vi "Resize DI Command Array.vi"(1 "Command in":T1={"Mode"=enum."Off", "Digital Input"=enum."Unused", "Default Profile Index"=0, "Cal Freq [Hz]"=0.0, "Cal Duration [s]"=0.0, "Cal Increment [s]"=0.0, "Cal Pulses"=0, "TMP Command Sequence"=[{"Duration [s]"=0.0, "Level"=FALSE, "Run/Stop"=FALSE, "Profile Index"=0}, {"Duration [s]"=0.0, "Level"=FALSE, "Run/Stop"=FALSE, "Profile Index"=0}, {"Duration [s]"=0.0, "Level"=FALSE, "Run/Stop"=FALSE, "Profile Index"=0}, {"Duration [s]"=0.0, "Level"=FALSE, "Run/Stop"=FALSE, "Profile Index"=0}, {"Duration [s]"=0.0, "Level"=FALSE, "Run/Stop"=FALSE, "Profile Index"=0}, {"Duration [s]"=0.0, "Level"=FALSE, "Run/Stop"=FALSE, "Profile Index"=0}, {"Duration [s]"=0.0, "Level"=FALSE, "Run/Stop"=FALSE, "Profile Index"=0}, {"Duration [s]"=0.0, "Level"=FALSE, "Run/Stop"=FALSE, "Profile Index"=0}], "EPT TDC Offset [CAD]"=0.0, "EPT Window Start [DBTDC]"=0.0, "EPT Window End [DBTDC]"=0.0, "EPT Angles"=[{"Enable"=FALSE, "Timing [DBTDC]"=0.0, "Duration [s]"=0.0, "Profile Index"=0}, {"Enable"=FALSE, "Timing [DBTDC]"=0.0, "Duration [s]"=0.0, "Profile Index"=0}, {"Enable"=FALSE, "Timing [DBTDC]"=0.0, "Duration [s]"=0.0, "Profile Index"=0}, {"Enable"=FALSE, "Timing [DBTDC]"=0.0, "Duration [s]"=0.0, "Profile Index"=0}], "EPT Skip Fire"=FALSE, "EPT Skip Index"=0, "EPT Precharge Duration [s]"=0.0, "EPT Precharge Profile Index"=0} {"EPT Precharge Profile Index" max=15; "EPT Precharge Duration [s]" min=0 format="%#_4p"; "Default Profile Index" max=15; "Cal Increment [s]" format="%#_3p"; "TMP Command Sequence"."Profile Index" max=7; "TMP Command Sequence"."Duration [s]" min=0 max=100 format="%#_3p"; "Cal Pulses" max=511; "EPT Skip Index" max=7; "EPT Angles"."Profile Index" max=7; "EPT Angles"."Duration [s]" min=0 max=100 format="%#_3p"; "Cal Duration [s]" format="%#_3p"; "Cal Freq [Hz]" format="%#_3p"}) -> (0 "Command out":T1={"Mode"=enum."Off", "Digital Input"=enum."Unused", "Default Profile Index"=0, "Cal Freq [Hz]"=0.0, "Cal Duration [s]"=0.0, "Cal Increment [s]"=0.0, "Cal Pulses"=0, "TMP Command Sequence"=[{"Duration [s]"=0.0, "Level"=FALSE, "Run/Stop"=FALSE, "Profile Index"=0}, {"Duration [s]"=0.0, "Level"=FALSE, "Run/Stop"=FALSE, "Profile Index"=0}, {"Duration [s]"=0.0, "Level"=FALSE, "Run/Stop"=FALSE, "Profile Index"=0}, {"Duration [s]"=0.0, "Level"=FALSE, "Run/Stop"=FALSE, "Profile Index"=0}, {"Duration [s]"=0.0, "Level"=FALSE, "Run/Stop"=FALSE, "Profile Index"=0}, {"Duration [s]"=0.0, "Level"=FALSE, "Run/Stop"=FALSE, "Profile Index"=0}, {"Duration [s]"=0.0, "Level"=FALSE, "Run/Stop"=FALSE, "Profile Index"=0}, {"Duration [s]"=0.0, "Level"=FALSE, "Run/Stop"=FALSE, "Profile Index"=0}], "EPT TDC Offset [CAD]"=0.0, "EPT Window Start [DBTDC]"=0.0, "EPT Window End [DBTDC]"=0.0, "EPT Angles"=[{"Enable"=FALSE, "Timing [DBTDC]"=0.0, "Duration [s]"=0.0, "Profile Index"=0}, {"Enable"=FALSE, "Timing [DBTDC]"=0.0, "Duration [s]"=0.0, "Profile Index"=0}, {"Enable"=FALSE, "Timing [DBTDC]"=0.0, "Duration [s]"=0.0, "Profile Index"=0}, {"Enable"=FALSE, "Timing [DBTDC]"=0.0, "Duration [s]"=0.0, "Profile Index"=0}], "EPT Skip Fire"=FALSE, "EPT Skip Index"=0, "EPT Precharge Duration [s]"=0.0, "EPT Precharge Profile Index"=0} {"EPT Precharge Profile Index" max=15; "EPT Precharge Duration [s]" min=0 format="%#_4p"; "Default Profile Index" max=15; "Cal Increment [s]" format="%#_3p"; "TMP Command Sequence"."Profile Index" max=7; "TMP Command Sequence"."Duration [s]" min=0 max=100 format="%#_3p"; "Cal Pulses" max=511; "EPT Skip Index" max=7; "EPT Angles"."Profile Index" max=7; "EPT Angles"."Duration [s]" min=0 max=100 format="%#_3p"; "Cal Duration [s]" format="%#_3p"; "Cal Freq [Hz]" format="%#_3p"})   [LabVIEW 2016]
uses:
  <vilib>/Powertrain Controls/Device Drivers/DCM/DI/RT/Command.ctl
  <vilib>/Powertrain Controls/Device Drivers/DCM/DI/FPGA/Mode.ctl
  <vilib>/Powertrain Controls/Device Drivers/DCM/Rev0/FPGA/Digital Channel.ctl
  <vilib>/Powertrain Controls/Device Drivers/DCM/DI/RT/Command Sequence.ctl
  <vilib>/Powertrain Controls/Device Drivers/DCM/DI/RT/Angle Control.ctl
  <vilib>/Powertrain Controls/Device Drivers/DCM/DI/RT/DCM - RT - DI.lvlib
  <vilib>/Powertrain Controls/Device Drivers/DCM/DI/FPGA/DCM - FPGA - DI.lvlib
  <vilib>/Powertrain Controls/Device Drivers/DCM/Rev0/FPGA/DCM - FPGA.lvlib
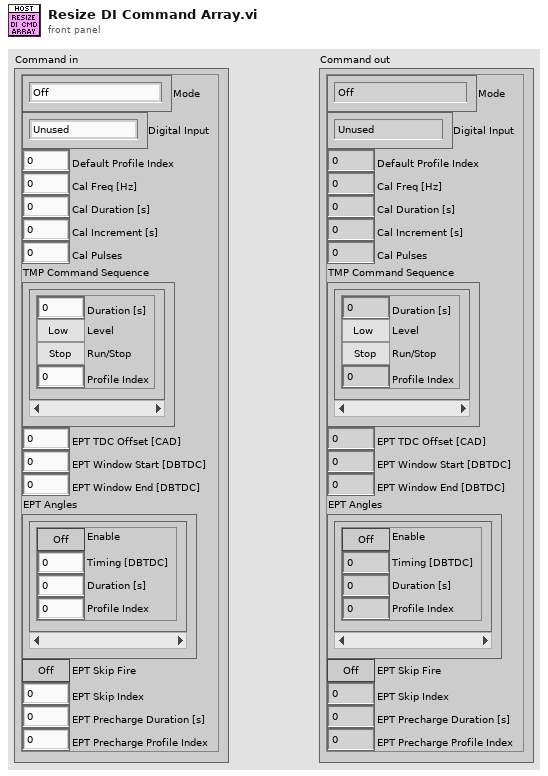
[diagram p1: front panel]
types:
  T1 = typedef "DCM - RT - DI.lvlib/Command.ctl" = cluster{"Mode":T2, "Digital Input":T3, "Default Profile Index":u8, "Cal Freq [Hz]":sgl, "Cal Duration [s]":sgl, "Cal Increment [s]":sgl, "Cal Pulses":u16, "TMP Command Sequence":T4[], "EPT TDC Offset [CAD]":sgl, "EPT Window Start [DBTDC]":sgl, "EPT Window End [DBTDC]":sgl, "EPT Angles":T5[], "EPT Skip Fire":bool, "EPT Skip Index":u8, "EPT Precharge Duration [s]":sgl, "EPT Precharge Profile Index":u8}
  T2 = typedef "DCM - FPGA - DI.lvlib/Mode.ctl" = enum8{"Off", "Direct", "Calibration", "Triggered Multi-Pulse", "Engine Position Tracking"}
  T3 = typedef "DCM - FPGA.lvlib/Digital Channel.ctl" = enum8{"Unused", "User OS", "Diff IO 1", "Diff IO 2", "Diff IO 3", "Diff IO 4", "Diff IO 5", "Diff IO 6", "Diff IO 7", "Diff IO 8", "Aux 1", "Aux 2", "Aux 3", "Aux 4", "Aux 5", "Aux 6", "Aux 7", "Aux 8", "Aux 9", "Aux 10", "Aux 11", "Aux 12", "Aux 13", "Aux 14", "Aux 15", "Aux 16"}
  T4 = typedef "DCM - RT - DI.lvlib/Command Sequence.ctl" = cluster{"Duration [s]":sgl, "Level":bool, "Run/Stop":bool, "Profile Index":u8}
  T5 = typedef "DCM - RT - DI.lvlib/Angle Control.ctl" = cluster{"Enable":bool, "Timing [DBTDC]":sgl, "Duration [s]":sgl, "Profile Index":u8}
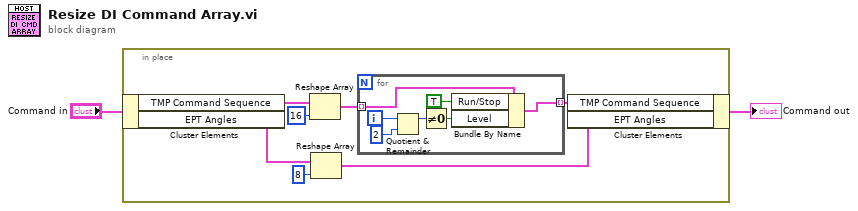
[diagram p0: block diagram]
diagram:
  n1 = in-place {
    n2 = in-place-cluster #1("Command in") -> ("TMP Command Sequence"=w6:T4[], "EPT Angles"=w9:T5[])
    n3 = Reshape Array(w6, 16 ("dimension size")) -> (w4:T4[])
    n4 = Reshape Array(w9, 8 ("dimension size")) -> (w8:T5[])
    n5 = for {
      tunnel: w4 -> [w16] mode=indexing
      tunnel: [w15] -> w3 mode=indexing
      i -> [w13]
      n6 = Quotient & Remainder(x=w13, y=2) -> (x-y*floor(x/y)=w11:i32)  [unwired: 1 out]
      n7 = Not Equal To 0?(x=w11) -> (x != 0?=w10:bool)
      n8 = Bundle By Name(cluster=w16, "Run/Stop"=TRUE ("Run"), "Level"=w10) -> (w15:T4)
    }
    n9 = in-place-cluster #1("TMP Command Sequence"=w3, "EPT Angles"=w8) -> (→"Command out":T1)
  }
